vi "FTW-Actor-HandleError.vi"(0 "FTW Actor Instance":refnum<class "FTW-ActorInstance.lvclass">, 5 "Explanation":string, 11 "error in":errorcluster) -> (4 "FTW Actor Instance out":refnum<class "FTW-ActorInstance.lvclass">, 6 "Exception occured?":T1, 15 "error out":errorcluster)   [LabVIEW 2012, in "FTW-Actor.lvlib" / "FTW-ActorInstance.lvclass"]
uses:
  FTW-ActorInstance.lvclass
  Core/Error/FTW-ERR-ExceptionType.ctl
panel:
  # "Inputs"
  # "Outputs"
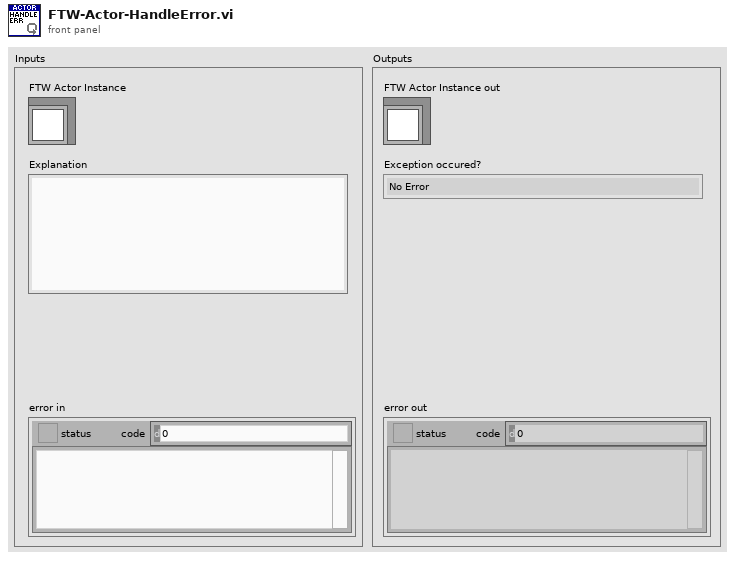
[diagram p1: front panel]
types:
  T1 = typedef "FTW-ERR-ExceptionType.ctl" = enum16{"No Error", "Error", "Warning"}
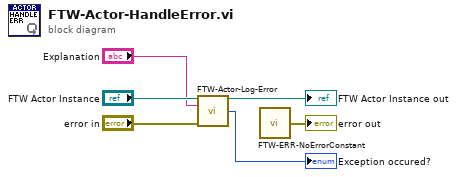
[diagram p0: block diagram]
diagram:
  n1 = call-dynamic "FTW-Actor-Log-Error.vi"("Featherweight Actor"="FTW Actor Instance", "Explanation"="Explanation", "Error to Log"="error in") -> ("Featherweight Actor out"=→"FTW Actor Instance out":refnum<class "FTW-ActorInstance.lvclass">, "Exception"=→"Exception occured?":T1)  [unwired: 9 in, 2 out]
  n2 = call "FTW-ERR-NoErrorConstant.vi"() -> ("no error"=→"error out":errorcluster)
